vi "ToArraySplit.vi"(8 "sortie d'erreur":errorcluster, 11 "Return value":string="['TRAIN:', [0, 1], 'TEST:', [2, 3], 'X_train:', [[1, 2], [3, 4]], 'X_test:', [[5, 6], [7, 8]], 'y_train:', [1, 2], 'y_test:', [3, 4], 'TRAIN:', [2, 3], 'TEST:', [0, 1], 'X_train:', [[5, 6], [7, 8]], 'X_test:', [[1, 2], [3, 4]], 'y_train:', [3, 4], 'y_test:', [1, 2]]") -> (0 "sortie d'erreur":errorcluster, 3 "Split":T1(array[cluster]))   [LabVIEW 2020]
uses:
  <vilib>/Utility/error.llb/Error Cluster From Error Code.vi
  <vilib>/ErrorRing/Error Ring.xnode
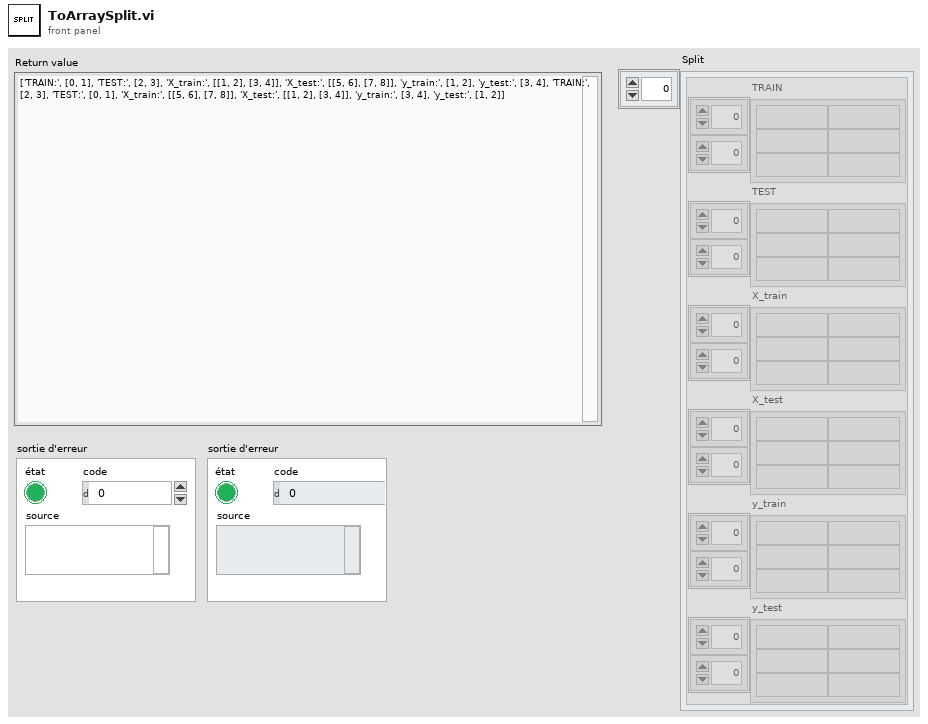
[diagram p1: front panel]
types:
  T1 = cluster{"TRAIN":string[][], "TEST":string[][], "X_train":string[][], "X_test":string[][], "y_train":string[][], "y_test":string[][]}[]
  T2 = cluster{"TRAIN":string[][], "TEST":string[][], "X_train":string[][], "X_test":string[][], "y_train":string[][], "y_test":string[][]}
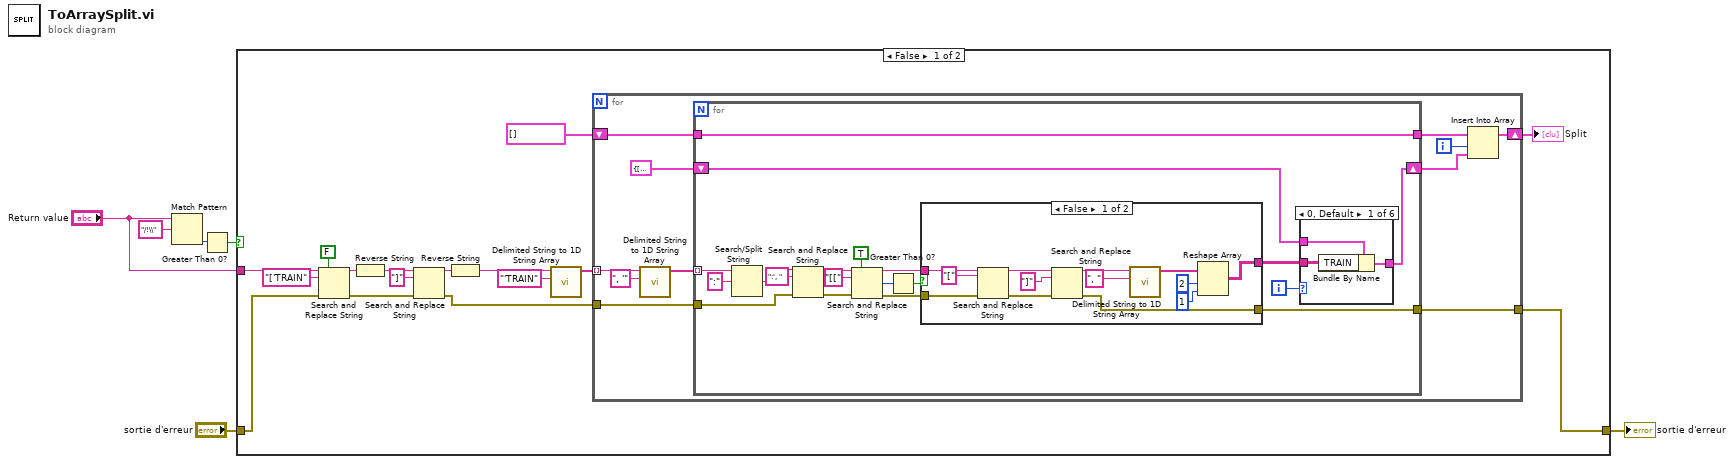
[diagram p0: block diagram]
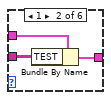
[diagram p2: hidden frame]
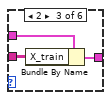
[diagram p3: hidden frame]
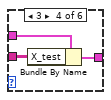
[diagram p4: hidden frame]
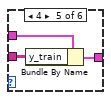
[diagram p5: hidden frame]
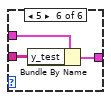
[diagram p6: hidden frame]
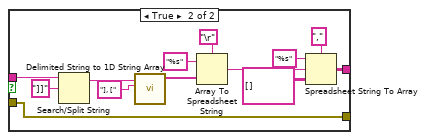
[diagram p7: hidden frame]
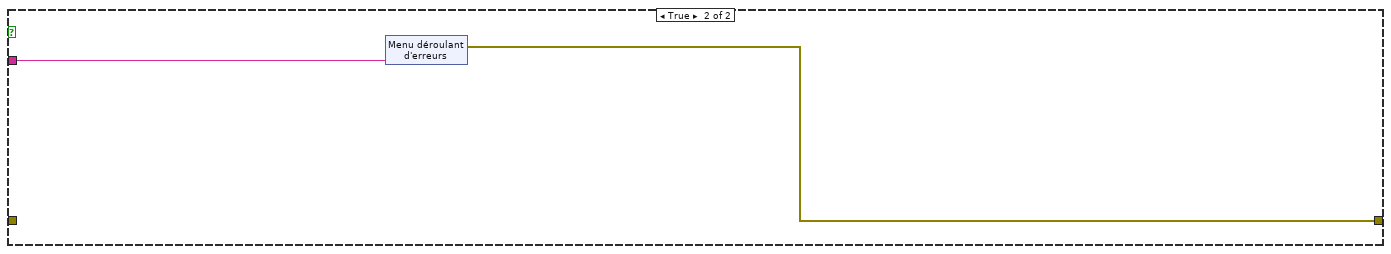
[diagram p8: hidden frame]
diagram:
  n1 = Match Pattern(string="Return value", regular expression="/!\\" ("expression régulière")) -> (offset past match=w5:i32)  [unwired: 1 in, 3 out]
  n2 = Greater Than 0?(x=w5) -> (x > 0?=w4:bool)
  n3 = case shown="False" w4 {
    tunnel: "Return value" -> [w22 w98]
    tunnel: [w9 w97] -> w3
    tunnel: "sortie d'erreur" -> [w12 _]
    frame False {
      n4 = Search and Replace String(replace all?=FALSE ("replace all? (F)"), input string=w22, search string="['TRAIN", error in=w12) -> (result string=w17:string, error out=w11:errorcluster)  [unwired: 4 in, 2 out]
      n5 = Reverse String(1:w17) -> (0:w16:string)
      n6 = Search and Replace String(input string=w16, search string="]", error in=w11) -> (result string=w14:string, error out=w10:errorcluster)  [unwired: 5 in, 2 out]
      n7 = Reverse String(1:w14) -> (0:w13:string)
      n8 = call <vilib>:"Delimited String to 1D String Array.vi"("delimiter"="'TRAIN", "delimited string"=w13) -> ("string array"=w18:string[])  [unwired: 9 in]
      n9 = for {
        tunnel: w18 -> [w32] mode=indexing
        tunnel: w10 -> [w30]
        tunnel: [w29] -> w9
        shift-right: [w25] -> w7
        shift-left: T1 [] ("Array") -> [w28]
        i -> [w26]
        n10 = call <vilib>:"Delimited String to 1D String Array.vi"("delimiter"=", '", "delimited string"=w32) -> ("string array"=w31:string[])  [unwired: 9 in]
        n11 = for {
          tunnel: w31 -> [w45] mode=indexing
          tunnel: w30 -> [w40]
          tunnel: [w46] -> w29
          tunnel: w28 -> [w38]
          tunnel: [w38] -> w27
          shift-right: [w35] -> w23
          shift-left: T2 {"TRAIN"=[], "TEST"=[], "X_train"=[], "X_test"=[], "y_train"=[], "y_test"=[]} ("Cluster") -> [w36]
          i -> [w37]
          n12 = Search/Split String(string=w45, search string/char (-)=":") -> (match + rest of string=w43:string)  [unwired: 1 in, 2 out]
          n13 = Search and Replace String(input string=w43, search string=":', ", error in=w40) -> (result string=w41:string, error out=w39:errorcluster)  [unwired: 5 in, 2 out]
          n14 = Search and Replace String(replace all?=TRUE ("replace all? (F)"), input string=w41, search string="[[", error in=w39) -> (result string=w48:string, number of replacements=w50:i32, error out=w47:errorcluster)  [unwired: 4 in, 1 out]
          n15 = Greater Than 0?(x=w50) -> (x > 0?=w49:bool)
          n16 = case shown="False" w49 {
            tunnel: w48 -> [w79 w93]
            tunnel: w47 -> [w77 w85]
            tunnel: [w75 w85] -> w46
            tunnel: [w71 w84] -> w34
            frame False {
              n17 = Search and Replace String(input string=w79, search string="[", error in=w77) -> (result string=w80:string, error out=w76:errorcluster)  [unwired: 5 in, 2 out]
              n18 = Search and Replace String(input string=w80, search string="]", error in=w76) -> (result string=w78:string, error out=w75:errorcluster)  [unwired: 5 in, 2 out]
              n19 = call <vilib>:"Delimited String to 1D String Array.vi"("delimiter"=", ", "delimited string"=w78) -> ("string array"=w74:string[])  [unwired: 9 in]
              n20 = Reshape Array(w74, 2 ("dimension size"), 1 ("dimension size")) -> (w71:string[][])
            }
            frame True {
              n21 = Search/Split String(string=w93, search string/char (-)="]]" ("chaîne/car. recherché (-)")) -> (substring before match=w92:string)  [unwired: 1 in, 2 out]
              n22 = call <vilib>:"Delimited String to 1D String Array.vi"("delimiter"="], [", "delimited string"=w92) -> ("string array"=w95:string[])  [unwired: 9 in]
              n23 = Array To Spreadsheet String(delimiter (Tab)="\r", array=w95, 3:"%s" ("chaîne de format")) -> (spreadsheet string=w86:string)
              n24 = Spreadsheet String To Array(delimiter (Tab)="," ("séparateur (Tabulation)"), format string="%s" ("chaîne de format"), spreadsheet string=w86, array type (2D Dbl)=string[][] []) -> (array=w84:string[][])
            }
          }
          n25 = case shown="0, Default" w37 {
            tunnel: w36 -> [w55 w58 w61 w64 w67 w70]
            tunnel: [w54 w57 w60 w63 w66 w69] -> w35
            tunnel: w34 -> [w53 w56 w59 w62 w65 w68]
            frame 0, Default {
              n26 = Bundle By Name(cluster=w55, "TRAIN"=w53) -> (w54:T2)
            }
            frame 1 {
              n27 = Bundle By Name(cluster=w58, "TEST"=w56) -> (w57:T2)
            }
            frame 2 {
              n28 = Bundle By Name(cluster=w61, "X_train"=w59) -> (w60:T2)
            }
            frame 3 {
              n29 = Bundle By Name(cluster=w64, "X_test"=w62) -> (w63:T2)
            }
            frame 4 {
              n30 = Bundle By Name(cluster=w67, "y_train"=w65) -> (w66:T2)
            }
            frame 5 {
              n31 = Bundle By Name(cluster=w70, "y_test"=w68) -> (w69:T2)
            }
          }
        }
        n32 = Insert Into Array(array=w27, index=w26, new element=w23) -> (w25:T1)
      }
      "Split" <- w7
    }
    frame True {
      n33 = xnode "Menu déroulant d'erreurs"("parameter 0"=w98) -> ("error out"=w97:errorcluster)
    }
  }
  "sortie d'erreur" <- w3
